vi "Auto Shot Routine.vi"(0 "Enable":bool, 1 "Speed to run intake motor (negated)":dbl=0.2, 5 "Time to wait after boulder out":u32, 9 "Wait for SpinUp":u32, 11 "Wait for Shot Time":u32) -> ()   [LabVIEW 2015]
uses:
  Robot Global Data.vi
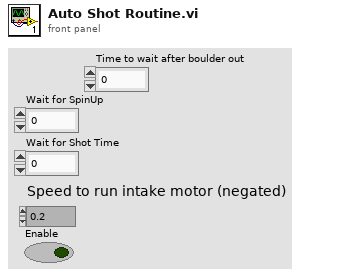
[diagram p1: front panel]
types:
  T1 = typedef "WPI_MotorControlDeviceRef.ctl" = cluster{"DeviceStatus":errorcluster, "Type":T2, "PWM":cluster{"PWM Channel":T3, "DeadBand":T4}, "CAN":cluster{"Device Number":u8, "Control Mode":T5, "Semaphore":T6, "Max Vout":dbl, "TalonSRX Control Mode":T7}, "Invert":bool}
  T2 = typedef "WPI_MotorControlType.ctl" = enum16{"PWM", "CAN", "CANTalonSRX"}
  T3 = typedef "FPGA_DIOPWMChannel.ctl" = enum8{"PWM 0", "PWM 1", "PWM 2", "PWM 3", "PWM 4", "PWM 5", "PWM 6", "PWM 7", "PWM 8", "PWM 9", "PWM MXP 0", "PWM MXP 1", "PWM MXP 2", "PWM MXP 3", "PWM MXP 4", "PWM MXP 5", "PWM MXP 6", "PWM MXP 7", "PWM MXP 8", "PWM MXP 9", "Invalid"}
  T4 = typedef "WPI_PWMDeadband.ctl" = cluster{"Name":string, "maxPositivePwm":i32, "minPositivePwm":i32, "centerPwm":i32, "maxNegativePwm":i32, "minNegativePwm":i32, "angularRange":u16}
  T5 = typedef "WPI_CANJaguar_ControlMode.ctl" = enum8{"Percent VBus", "Current", "Speed", "Position", "Voltage"}
  T6 = typedef "Semaphore RefNum" = refnum<k1>
  T7 = typedef "WPI_CANTalonSRX_APIControlMode.ctl" = enum8{"Percent VBus", "Speed", "Position", "Slave", "Unchanged / Invalid", "Voltage Compensation", "Current", "Motion Profile"}
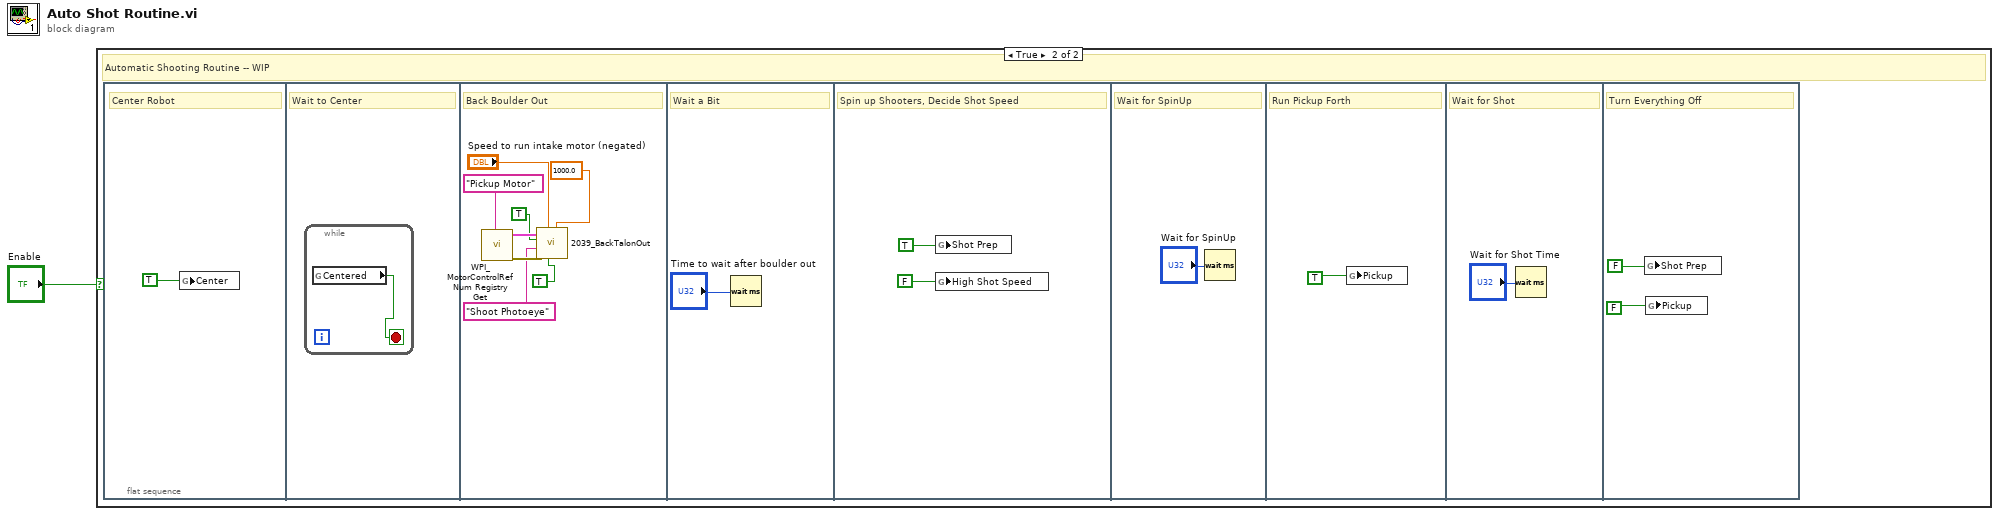
[diagram p0: block diagram]
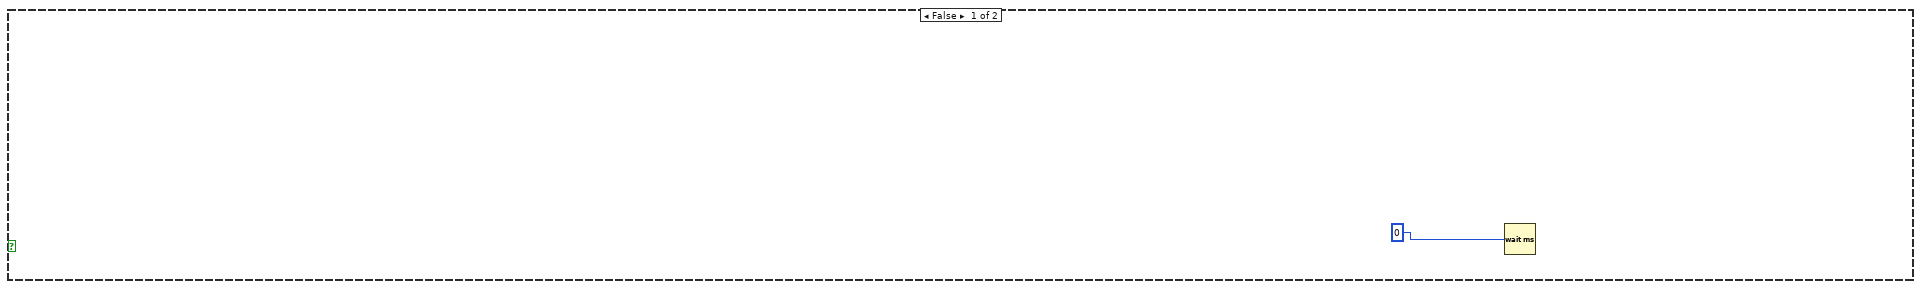
[diagram p2: hidden frame]
diagram:
  n1 = case shown="True" "Enable" {
    frame False {
      n2 = Wait (ms)(milliseconds to wait=u32 0) -> ()  [unwired: 1 out]
    }
    frame True {
      # "Automatic Shooting Routine -- WIP"
      n3 = flat-sequence {
        frame #0 {
          # "Center Robot"
          n4 = global write "Robot Global Data.vi" "Center"(TRUE) -> ()
        }
        frame #1 {
          # "Wait to Center"
          n5 = while {
            stop <- w4 stop-if-true
            n6 = global read "Robot Global Data.vi" "Centered"() -> (w4:bool)
          }
        }
        frame #2 {
          # "Back Boulder Out"
          n7 = call <vilib>:"WPI_MotorControlRefNum Registry Get.vi"("refnum name"="Pickup Motor") -> ("error out"=w12:errorcluster, "MotorControlDevRef"=w11:T1)  [unwired: 9 in]
          n8 = call "2039_BackTalonOut.vi"("Throttle Ramp Rate (percent/s)"=1000.0, "Invert Stop Condition"=TRUE, "Speed to run motor (will be negated)"="Speed to run intake motor (negated)", "error in (no error)"=w12, "DIO Ref Name"="Shoot Photoeye", "Brake"=TRUE, "CAN Talon SRX Ref"=w11) -> ()  [unwired: 3 in, 2 out]
        }
        frame #3 {
          # "Wait a Bit"
          n9 = Wait (ms)(milliseconds to wait="Time to wait after boulder out") -> ()  [unwired: 1 out]
        }
        frame #4 {
          # "Spin up Shooters, Decide Shot Speed"
          n10 = global write "Robot Global Data.vi" "Shot Prep"(TRUE) -> ()
          n11 = global write "Robot Global Data.vi" "High Shot Speed"(FALSE) -> ()
        }
        frame #5 {
          # "Wait for SpinUp"
          n12 = Wait (ms)(milliseconds to wait="Wait for SpinUp") -> ()  [unwired: 1 out]
        }
        frame #6 {
          # "Run Pickup Forth"
          n13 = global write "Robot Global Data.vi" "Pickup"(TRUE) -> ()
        }
        frame #7 {
          # "Wait for Shot"
          n14 = Wait (ms)(milliseconds to wait="Wait for Shot Time") -> ()  [unwired: 1 out]
        }
        frame #8 {
          # "Turn Everything Off"
          n15 = global write "Robot Global Data.vi" "Shot Prep"(FALSE) -> ()
          n16 = global write "Robot Global Data.vi" "Pickup"(FALSE) -> ()
        }
      }
    }
  }
